vi "Open-Close Items.vi"(8 "error in (no error)":errorcluster, 9 "Tag (\"\")":string, 10 "Action (Close All)":T1=enum."Close All", 11 "Tree in":refnum<class "TreeControl.lvclass">) -> (0 "error out":errorcluster, 3 "Tree (dup)":refnum<class "TreeControl.lvclass">)   [LabVIEW 2015, in "TreeControl.lvclass"]
doc: "<b> </b> <b> </b>\n©2016 Q Software Innovations, LLC (QSI)\nwritten by Quentin Alldredge\nproduced in LabVIEW 2015\n\nsupport@qsoftwareinnovations.com\nwww.qsoftwareinnovations.com\n\nAll rights reserved.\n\nRedistribution and use in source and binary forms, with or without modification, are permitted provided that the following conditions are met:\n\n * Redistributions of source code must retain the above copyright notice, this list of conditions and the following disclaimer.\n * Redistributions in binary form must reproduce the above copyright notice, this list of conditions and the following disclaimer in the documentation and/or other materials provided with the distribution.\n * Neither the name of Q Software Innovations, LLC. nor the names of its contributors may be used to endorse or promote products derived from this software without specific prior written permission.\n\nTHIS SOFTWARE IS PROVIDED BY THE COPYRIGHT HOLDERS AND CONTRIBUTORS \"AS IS\" AND ANY EXPRESS OR IMPLIED WARRANTIES, INCLUDING, BUT NOT LIMITED TO, THE IMPLIED WARRANTIES OF MERCHANTABILITY AND FITNESS FOR A PARTICULAR PURPOSE ARE DISCLAIMED. IN NO EVENT SHALL THE COPYRIGHT OWNER OR CONTRIBUTORS BE LIABLE FOR ANY DIRECT, INDIRECT, INCIDENTAL, SPECIAL, EXEMPLARY, OR CONSEQUENTIAL DAMAGES (INCLUDING, BUT NOT LIMITED TO, PROCUREMENT OF SUBSTITUTE GOODS OR SERVICES; LOSS OF USE, DATA, OR PROFITS; OR BUSINESS INTERRUPTION) HOWEVER CAUSED AND ON ANY THEORY OF LIABILITY, WHETHER IN CONTRACT, STRICT LIABILITY, OR TORT (INCLUDING NEGLIGENCE OR OTHERWISE) ARISING IN ANY WAY OUT OF THE USE OF THIS SOFTWARE, EVEN IF ADVISED OF THE POSSIBILITY OF SUCH DAMAGE."
uses:
  TreeControl.lvclass
  Tree Action Enum.ctl
  TreeControl.lvclass/TreeControl.ctl
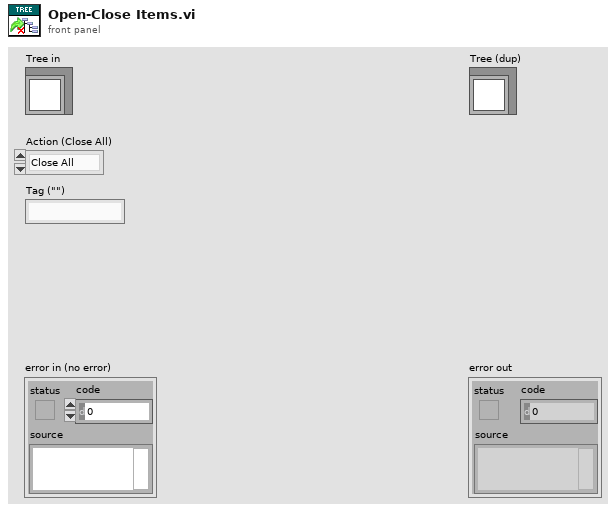
[diagram p1: front panel]
types:
  T1 = typedef "TreeControl.lvclass/Tree Action Enum.ctl" = enum16{"Open All", "Close All", "Open Item", "Close Item"}
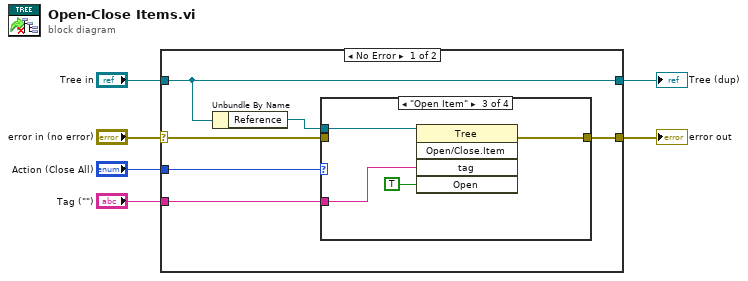
[diagram p0: block diagram]
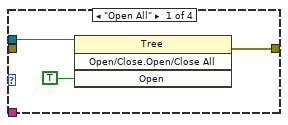
[diagram p2: hidden frame]
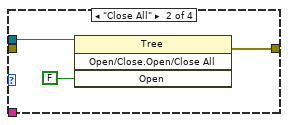
[diagram p3: hidden frame]
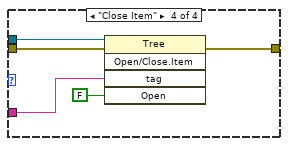
[diagram p4: hidden frame]
diagram:
  n1 = case shown="No Error" "error in (no error)" {
    selector: "error in (no error)" -> [w9 w29]
    tunnel: [w12 w29] -> w5
    tunnel: [w8 w28] -> w3
    tunnel: "Tree in" -> [w8 w28]
    tunnel: "Action (Close All)" -> [w11 _]
    tunnel: "Tag (\"\")" -> [w10 _]
    frame No Error {
      n2 = Unbundle By Name(w8) -> ("Reference"=w7:refnum<vi>)
      n3 = case shown="\"Open Item\"" w11 {
        tunnel: w7 -> [w15 w18 w22 w27]
        tunnel: [w13 w16 w19 w24] -> w12
        tunnel: w10 -> [_ _ w21 w26]
        tunnel: w9 -> [_ _ _ w23]
        frame "Open All" {
          n4 = invoke class="Tree" method="Open/Close.Open/Close All"(reference=w15, "Open"=TRUE ("Open?")) -> (error out=w13:errorcluster)  [unwired: 2 in, 3 out]
        }
        frame "Close All" {
          n5 = invoke class="Tree" method="Open/Close.Open/Close All"(reference=w18, "Open"=FALSE ("Open?")) -> (error out=w16:errorcluster)  [unwired: 2 in, 3 out]
        }
        frame "Open Item" {
          n6 = invoke class="Tree" method="Open/Close.Item"(reference=w22, "tag"=w21, "Open"=TRUE ("Open?")) -> (error out=w19:errorcluster)  [unwired: 2 in, 4 out]
        }
        frame "Close Item" {
          n7 = invoke class="Tree" method="Open/Close.Item"(reference=w27, error in=w23, "tag"=w26, "Open"=FALSE ("Open?")) -> (error out=w24:errorcluster)  [unwired: 1 in, 4 out]
        }
      }
    }
    frame Error {
    }
  }
  "error out" <- w5
  "Tree (dup)" <- w3
